vi "USB Retry Connect.vi"(11 "DevHandle":i32) -> (3 "function return":u8)   [LabVIEW 2010, in "usb_device.lvlib"]
doc: "unsigned char WINAPI USB_RetryConnect(int DevHandle);"
uses:
  usb_device.lvlib
  USB2XXX/trunk/USB2XXX/USB2XXX/vs2019/Release/USB2XXX.dll
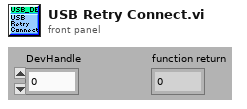
[diagram p1: front panel]
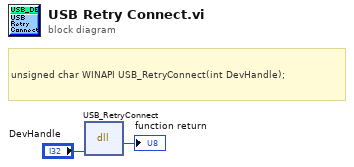
[diagram p0: block diagram]
diagram:
  # "unsigned char WINAPI USB_RetryConnect(int DevHandle);"
  n1 = dll-call lib="E:/Projects/USB2XXX/trunk/USB2XXX/USB2XXX/vs2019/Release/USB2XXX.*" fn="USB_RetryConnect"("DevHandle"="DevHandle") -> (→"function return":u8)  [unwired: 4 in, 2 out]
